vi "UserInterfaceEventPattern.vi"() -> ()   [LabVIEW 2023]
doc: "Use this template to build a user interface event handler design pattern. Use this pattern for dialog boxes and other user interfaces. You also can create and execute user-defined events that the VI can handle the same way as user interface events."
panel:
  in  "Table":bool
  in  "Graph":bool
  in  "6@49":bool
  in  "stop":bool
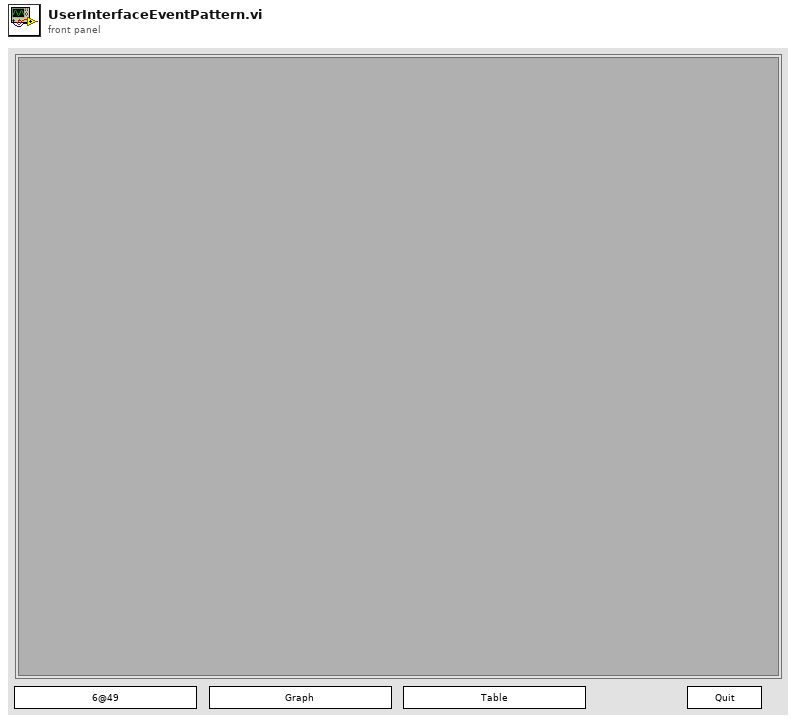
[diagram p1: front panel]
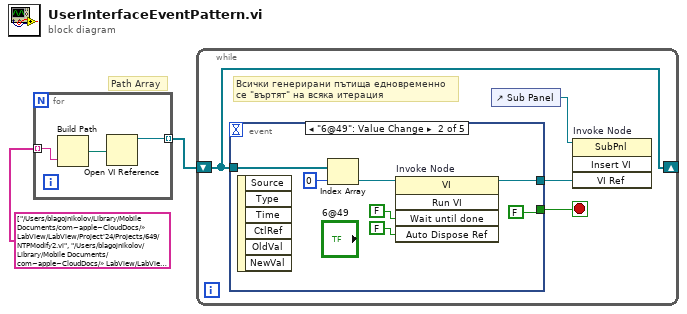
[diagram p0: block diagram]
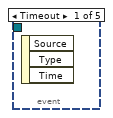
[diagram p2: hidden frame]
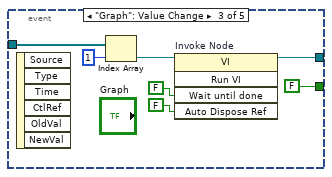
[diagram p3: hidden frame]
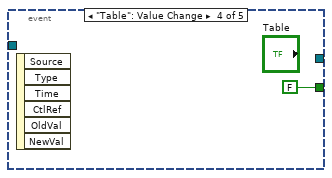
[diagram p4: hidden frame]
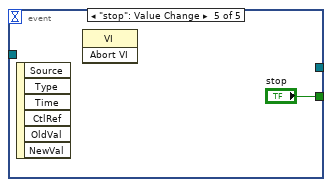
[diagram p5: hidden frame]
diagram:
  # "Path Array"
  n1 = for {
    tunnel: string[] ["/Users/blagojnikolov/Library/Mobile Documents/com~apple~CloudDocs/» LabView/LabView/Project'24/Projects/649/NTPModify2.vi", "/Users/blagojnikolov/Library/Mobile Documents/com~apple~CloudDocs/» LabView/LabView/Project'24/Projects/649/subVI Tools/StdsWaveforms.vi", "/Users/blagojnikolov/Library/Mobile Documents/com~apple~CloudDocs/» LabView/LabView/Project'24/Projects/649/subVI Tools/TableFormat.vi"] -> [w4] mode=indexing
    tunnel: [w3] -> w1 mode=indexing
    n2 = Build Path(name or relative path=w4) -> (appended path=w5:path)  [unwired: 1 in]
    n3 = Open VI Reference(vi path=w5) -> (vi reference=w3:refnum<vi>)  [unwired: 5 in, 1 out]
  }
  n4 = while {
    shift-right: [w8] -> _
    shift-left: w1 -> [w8]
    stop <- w9 stop-if-true
    # "Всички генерирани пътища едновременно\nсе \"въртят\" на всяка итерация"
    n5 = event shown="[1] \"6@49\": Value Change" {
      selector: _ -> [_ _ _ _ _]
      dyn-events: _ -> [_ _ _ _ _]
      timeout: _ -> [_ _ _ _ _]
      tunnel: [_ FALSE FALSE FALSE "stop"] -> w9
      tunnel: w8 -> [_ w14 w19 _ _]
      tunnel: [_ w11 w18 _ _] -> w6
      event Timeout {
        n6 = event-data() -> ()  [unwired: 1 in, 3 out]
      }
      event "6@49": Value Change {
        n7 = event-data() -> ()  [unwired: 1 in, 6 out]
        n8 = Index Array "Index Array"(array=w14, index=0) -> (element=w12:refnum<vi>)
        n9 = invoke on="Invoke Node" class="VI" method="Run VI"(reference=w12, "Wait until done"=FALSE ("Wait Until Done"), "Auto Dispose Ref"=FALSE ("Auto Dispose Reference")) -> (reference out=w11:refnum<vi>)  [unwired: 2 in, 4 out]
      }
      event "Graph": Value Change {
        n10 = event-data() -> ()  [unwired: 1 in, 6 out]
        n11 = Index Array "Index Array"(array=w19, index=1) -> (element=w20:refnum<vi>)
        n12 = invoke on="Invoke Node" class="VI" method="Run VI"(reference=w20, "Wait until done"=FALSE ("Wait Until Done"), "Auto Dispose Ref"=FALSE ("Auto Dispose Reference")) -> (reference out=w18:refnum<vi>)  [unwired: 2 in, 4 out]
      }
      event "Table": Value Change {
        n13 = event-data() -> ()  [unwired: 1 in, 6 out]
      }
      event "stop": Value Change {
        n14 = event-data() -> ()  [unwired: 1 in, 6 out]
        n15 = invoke class="VI" method="Abort VI"() -> ()  [unwired: 3 in, 3 out]
      }
    }
    n16 = control-ref of="Sub Panel"() -> (w7:refnum<vi>)
    n17 = invoke on="Invoke Node" class="SubPnl" method="Insert VI"(reference=w7, "VI Ref"=w6) -> ()  [unwired: 2 in, 4 out]
  }
